vi "Read Automotive Simulated Data.vi"(7 "Power Button":bool, 9 "Gear":i32(slide) scale=-1.0..5.0, 10 "Break":bool, 11 "Accelerator":bool) -> (0 "Temperature":dbl, 1 "Fuel Gauge":dbl, 2 "RPM":dbl, 3 "Speed":dbl, 5 "ON":bool)   [LabVIEW 2020]
uses:
  <vilib>/numeric/Random Number (Range) DBL.vi
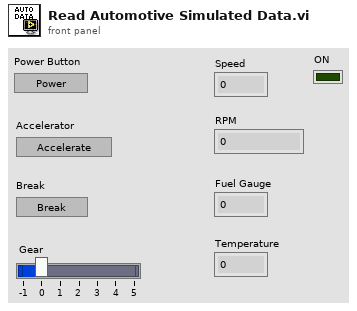
[diagram p1: front panel]
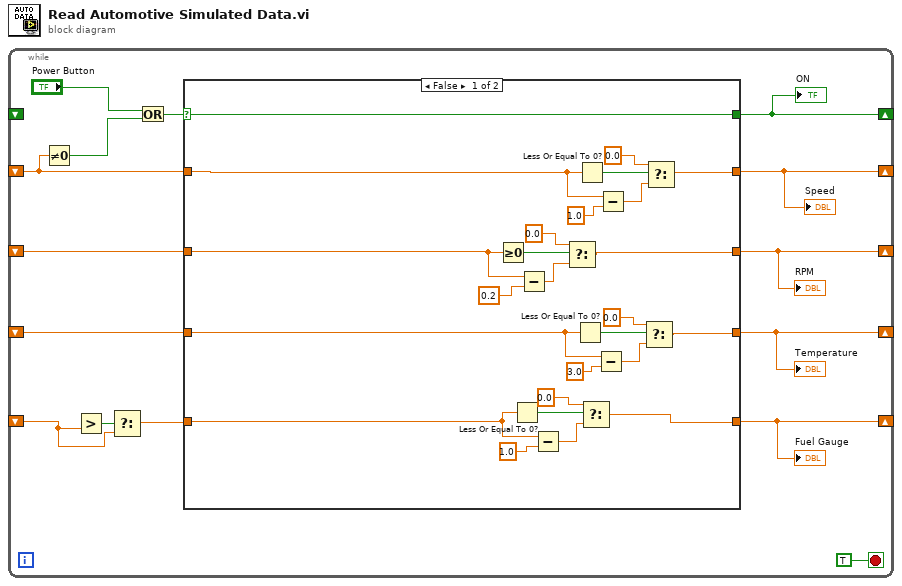
[diagram p0: block diagram]
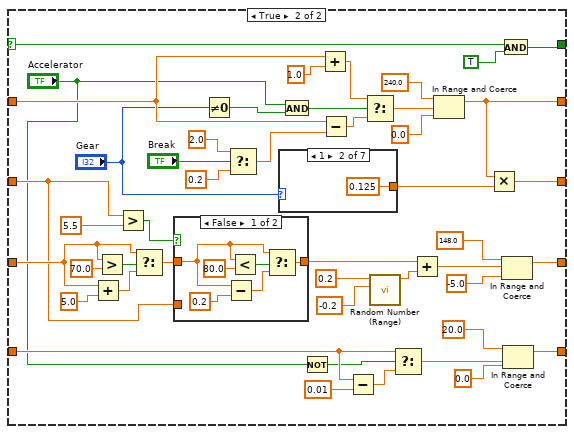
[diagram p2: hidden frame]
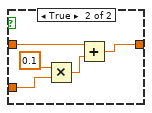
[diagram p3: hidden frame]
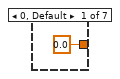
[diagram p4: hidden frame]
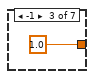
[diagram p5: hidden frame]
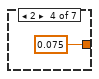
[diagram p6: hidden frame]
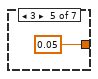
[diagram p7: hidden frame]
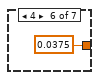
[diagram p8: hidden frame]
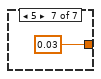
[diagram p9: hidden frame]
diagram:
  n1 = while {
    shift-right: [w7] -> _
    shift-left: _ -> [_]
    shift-right: [w12] -> _
    shift-left: _ -> [w10]
    shift-right: [w5] -> _
    shift-left: _ -> [w11]
    shift-right: [w13] -> _
    shift-left: _ -> [w2]
    shift-right: [w14] -> _
    shift-left: _ -> [w4]
    stop <- TRUE stop-if-true
    n2 = Not Equal To 0?(x=w10) -> (x != 0?=w9:bool)
    n3 = Greater?(y=w2) -> (0:w3:bool)  [unwired: 1 in]
    n4 = Select(s=w3, f=w2) -> (s? t:f=w1:dbl)  [unwired: 1 in]
    n5 = Or(x="Power Button", y=w9) -> (x .or. y?=w8:bool)
    n6 = case shown="False" w8 {
      selector: w8 -> [w20 w69]
      tunnel: [w21 w71] -> w12
      tunnel: [w31 w55] -> w5
      tunnel: [w39 w48] -> w13
      tunnel: [w26 w72] -> w14
      tunnel: w10 -> [w22 w81]
      tunnel: w11 -> [w32 w60]
      tunnel: w1 -> [w38 w44]
      tunnel: w4 -> [w27 w47]
      tunnel: [w20 w68] -> w7
      frame False {
        n7 = Greater Or Equal To 0?(x=w27) -> (x >= 0?=w30:bool)
        n8 = Less Or Equal To 0?(x=w38) -> (x <= 0?=w40:bool)
        n9 = Subtract(x=w27, y=0.2) -> (x-y=w29:dbl)
        n10 = Subtract(x=w38, y=1.0) -> (x-y=w37:dbl)
        n11 = Select(t=0.0, s=w30, f=w29) -> (s? t:f=w26:dbl)
        n12 = Less Or Equal To 0?(x=w32) -> (x <= 0?=w35:bool)
        n13 = Less Or Equal To 0?(x=w22) -> (x <= 0?=w25:bool)
        n14 = Select(t=0.0, s=w40, f=w37) -> (s? t:f=w39:dbl)
        n15 = Subtract(x=w32, y=3.0) -> (x-y=w34:dbl)
        n16 = Subtract(x=w22, y=1.0) -> (x-y=w24:dbl)
        n17 = Select(t=0.0, s=w35, f=w34) -> (s? t:f=w31:dbl)
        n18 = Select(t=0.0, s=w25, f=w24) -> (s? t:f=w21:dbl)
      }
      frame True {
        n19 = Add(x=w60, y=5.0) -> (x+y=w59:dbl)
        n20 = Greater?(x=w60, y=70.0 ("f")) -> (0:w63:bool)
        n21 = Greater?(x=w47, y=5.5) -> (0:w66:bool)
        n22 = Select(t=w60, s=w63, f=w59) -> (s? t:f=w62:dbl)
        n23 = case shown="False" w66 {
          tunnel: w62 -> [w88 w97]
          tunnel: [w87 w96] -> w64
          tunnel: w47 -> [_ w93]
          frame False {
            n24 = Subtract(x=w88, y=0.2) -> (x-y=w92:dbl)
            n25 = Less?(x=w88, y=80.0 ("f")) -> (x < y?=w91:bool)
            n26 = Select(t=w88, s=w91, f=w92) -> (s? t:f=w87:dbl)
          }
          frame True {
            n27 = Multiply(x=0.1 ("y"), y=w93) -> (x*y=w95:dbl)
            n28 = Add(x=w97, y=w95) -> (x+y=w96:dbl)
          }
        }
        n29 = Not Equal To 0?(x="Gear") -> (x != 0?=w75:bool)
        n30 = Select(t=2.0, s="Break", f=0.2) -> (s? t:f=w77:dbl)
        n31 = case shown="1" "Gear" {
          tunnel: [0.0 0.125 1.0 0.075 0.05 0.0375 0.03] -> w70
          frame 0, Default {
          }
          frame 1 {
          }
          frame -1 {
          }
          frame 2 {
          }
          frame 3 {
          }
          frame 4 {
          }
          frame 5 {
          }
        }
        n32 = And(x="Accelerator", y=w75) -> (x .and. y?=w76:bool)
        n33 = Not(x="Accelerator") -> (.not. x?=w41:bool)
        n34 = Add(x=w81, y=1.0) -> (x+y=w83:dbl)
        n35 = Subtract(x=w81, y=w77) -> (x-y=w80:dbl)
        n36 = Subtract(x=w44, y=0.01) -> (x-y=w45:dbl)
        n37 = Select(t=w83, s=w76, f=w80) -> (s? t:f=w73:dbl)
        n38 = call-poly <vilib>:"Random Number (Range).vi"("lower bound (0)"=-0.2, "upper bound (100)"=0.2) -> ("number"=w53:dbl)  [unwired: 9 in]
        n39 = Select(t=w44, s=w41, f=w45) -> (s? t:f=w43:dbl)
        n40 = Add(x=w64, y=w53) -> (x+y=w54:dbl)
        n41 = In Range and Coerce(upper limit=240.0, x=w73, lower limit=0.0) -> (coerced(x)=w71:dbl)  [unwired: 1 out]
        n42 = Multiply(x=w71, y=w70) -> (x*y=w72:dbl)
        n43 = And(x=w69, y=TRUE) -> (x .and. y?=w68:bool)
        n44 = In Range and Coerce(upper limit=148.0, x=w54, lower limit=-5.0) -> (coerced(x)=w55:dbl)  [unwired: 1 out]
        n45 = In Range and Coerce(upper limit=20.0, x=w43, lower limit=0.0) -> (coerced(x)=w48:dbl)  [unwired: 1 out]
      }
    }
    "Speed" <- w12
    "Fuel Gauge" <- w13
    "Temperature" <- w5
    "RPM" <- w14
    "ON" <- w7
  }
